vi "Conveyor and Shooter SS Safety.vi"(11 "Conveyor and Shooter Actuator Values In":T1) -> (3 "Conveyor and Shooter Actuator Values Out":T1)   [LabVIEW 2016]
uses:
  Conveyor and Shooter Actuator Out.ctl
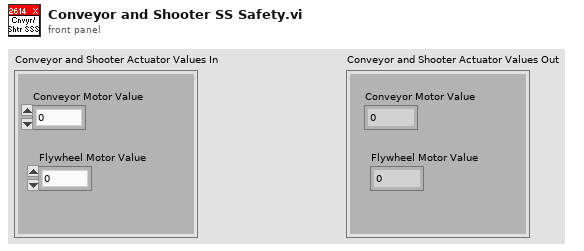
[diagram p1: front panel]
types:
  T1 = typedef "Conveyor and Shooter Actuator Out.ctl" = cluster{"Conveyor Motor Value":dbl, "Flywheel Motor Value":dbl}
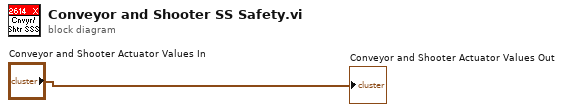
[diagram p0: block diagram]
diagram:
  "Conveyor and Shooter Actuator Values Out" <- "Conveyor and Shooter Actuator Values In"
